vi "pll_proba_diag_realtime.vi"(0 "all rows":dbl[][](array[numeric])=array100002x3[300006 elements] format="%0.5f", 5 "Resolution":dbl, 7 "t_ref":dbl[](array[numeric]), 9 "dt":dbl, 11 "Error In":errorcluster, 12 "Second":bool) -> (3 "average":dbl=2.3596690204414683, 4 "XY Graph":cluster{"all rows":dbl[], "all rows":dbl[]}[](graph), 6 "Waveform Graph":cluster{"f0":dbl, "df":dbl, "magnitude":dbl[]}(graph), 8 "time":dbl[](array[numeric]), 10 "Waveform Graph 2":cluster{"f0":dbl, "df":dbl, "magnitude":dbl[]}(graph), 13 "PLL_sine":dbl[](array[numeric]), 14 "PLL_cosine":dbl[](array[numeric]), 15 "Error Out":errorcluster)   [LabVIEW 2013]
uses:
  <vilib>/express/express analysis/Spectral/Block/exnSpectralBlock spectral measurements RMS poly.vi
  <vilib>/express/express analysis/Spectral/Block/exnSpectralBlock spectral measurements RMS WFM.vi
  <vilib>/express/express analysis/Spectral/XNode/ExpressSpectralMeasurementsBlockNode.xnode
panel:
  out "XY Graph 2":cluster{"all rows":dbl[], "all rows":dbl[]}[](graph)
  out "t_i-1":dbl
  out "t_i":dbl
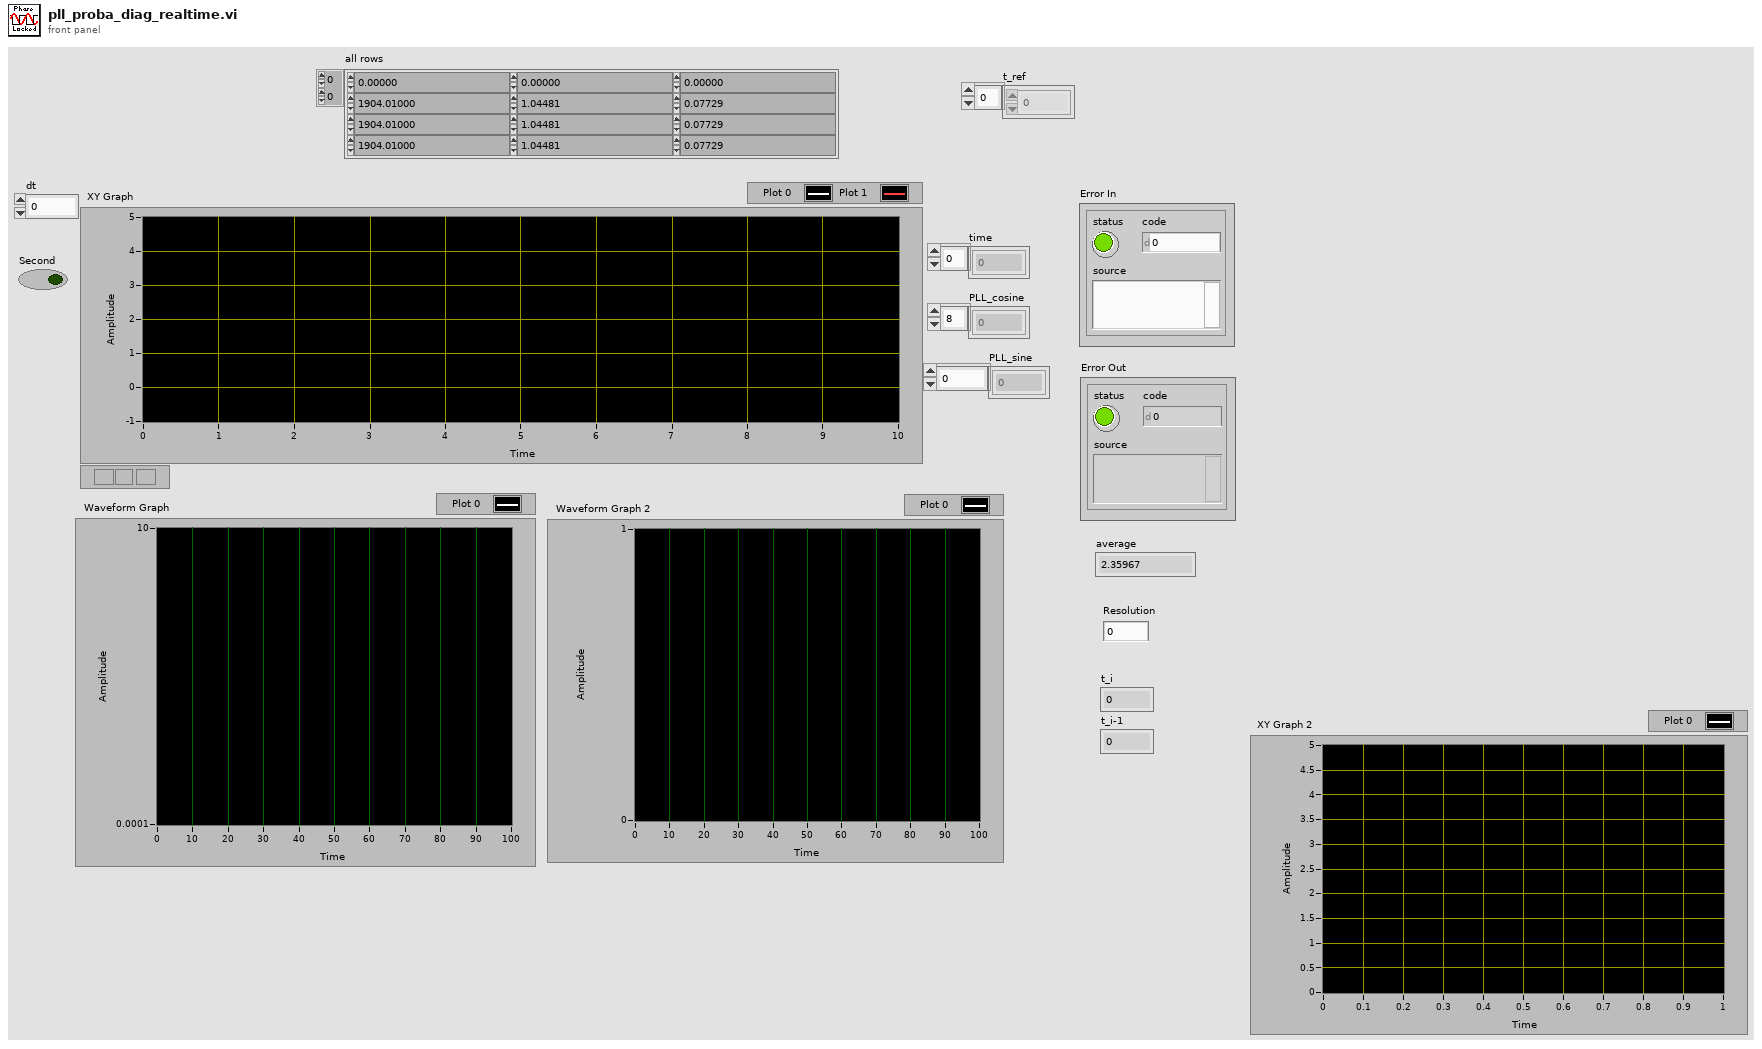
[diagram p1: front panel]
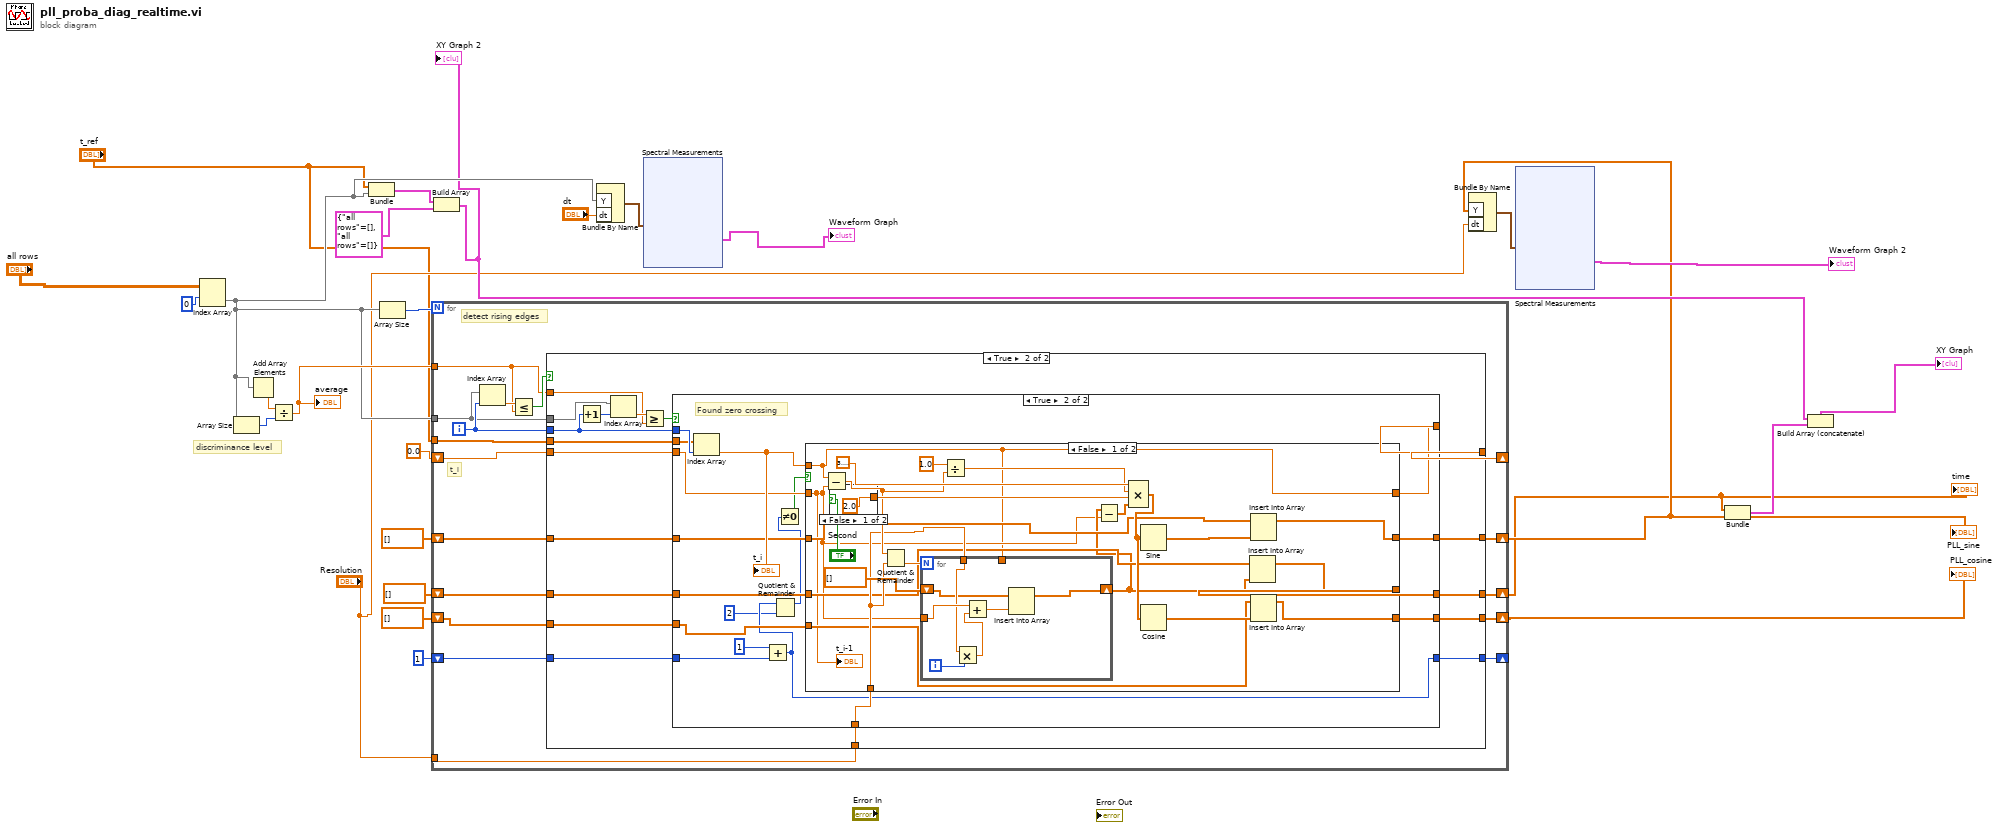
[diagram p0: block diagram]
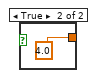
[diagram p4: hidden frame]
diagram:
  # "discriminance level"
  n1 = Index Array(array="all rows", index (row)=0 ("disabled index (col)")) -> (element=w19:dbl[])  [unwired: 1 in]
  n2 = Array Size(array=w19) -> (size(s)=w25:i32)
  n3 = Add Array Elements(numeric array=w19) -> (sum=w26:dbl)
  n4 = Divide(x=w26, y=w25) -> (x/y=w24:dbl)
  "average" <- w24
  n5 = Bundle("t_ref"="t_ref", "all rows"=w19) -> (w15:cluster{"t_ref":dbl[], "all rows":dbl[]})  [unwired: 1 in]
  n6 = Array Size(array=w19) -> (size(s)=w23:i32)
  n7 = for {
    N: w23 -> [_]
    tunnel: w19 -> [w42]
    tunnel: w24 -> [w40]
    tunnel: "t_ref" -> [w39]
    shift-right: [w38] -> _
    shift-left: 0.0 -> [w37]
    tunnel: "Resolution" -> [w36]
    shift-right: [w35] -> w5
    shift-left: dbl[] [] -> [w34]
    shift-right: [w33] -> w4
    shift-left: dbl[] [] -> [w32]
    shift-right: [w31] -> w3
    shift-left: dbl[] [] -> [w30]
    shift-right: [w29] -> _
    shift-left: 1 -> [w28]
    i -> [w43]
    # "t_i"
    # "detect rising edges"
    n8 = Index Array(array=w42, index=w43) -> (element=w41:dbl)
    n9 = Less Or Equal?(x=w41, y=w40) -> (x <= y?=w44:bool)
    n10 = case shown="True" w44 {
      tunnel: w43 -> [_ w61]
      tunnel: w42 -> [_ w67]
      tunnel: w40 -> [_ w63]
      tunnel: w39 -> [_ w62]
      tunnel: [w49 w60] -> w38
      tunnel: w37 -> [w49 w59]
      tunnel: w36 -> [_ w58]
      tunnel: [w48 w57] -> w35
      tunnel: w34 -> [w48 w56]
      tunnel: [w47 w55] -> w33
      tunnel: w32 -> [w47 w54]
      tunnel: [w46 w53] -> w31
      tunnel: w30 -> [w46 w52]
      tunnel: [w45 w51] -> w29
      tunnel: w28 -> [w45 w50]
      frame False {
      }
      frame True {
        n11 = Increment(x=w61) -> (x+1=w66:i32)
        n12 = Index Array(array=w67, index=w66) -> (element=w64:dbl)
        n13 = Greater Or Equal?(x=w64, y=w63) -> (x >= y?=w65:bool)
        n14 = case shown="True" w65 {
          tunnel: w62 -> [_ w89]
          tunnel: w61 -> [_ w90]
          tunnel: [w72 w73] -> w60
          tunnel: w59 -> [w72 w86]
          tunnel: w58 -> [_ w87]
          tunnel: [w71 w85] -> w57
          tunnel: w56 -> [w71 w82]
          tunnel: [w70 w84] -> w55
          tunnel: w54 -> [w70 w81]
          tunnel: [w69 w83] -> w53
          tunnel: w52 -> [w69 w80]
          tunnel: [w68 w77] -> w51
          tunnel: w50 -> [w68 w78]
          frame False {
          }
          frame True {
            # "Found zero crossing"
            n15 = Index Array(array=w89, index=w90) -> (element=w88:dbl)
            "t_i" <- w88
            n16 = Add(x=1, y=w78) -> (x+y=w77:i32)
            n17 = Quotient & Remainder(x=w77, y=2) -> (x-y*floor(x/y)=w74:i32)  [unwired: 1 out]
            n18 = Not Equal To 0?(x=w74) -> (x != 0?=w75:bool)
            n19 = case shown="False" w75 {
              tunnel: w86 -> [w92 w122]
              tunnel: w88 -> [w91 _]
              tunnel: w87 -> [w105 _]
              tunnel: [w97 w124] -> w84
              tunnel: [w100 w125] -> w85
              tunnel: [w94 w123] -> w83
              tunnel: w82 -> [w102 w125]
              tunnel: w81 -> [w99 w124]
              tunnel: w80 -> [w95 w123]
              tunnel: [w91 w122] -> w73
              frame False {
                n20 = Subtract(x=w91, y=w92) -> (x-y=w106:dbl)
                n21 = case shown="False" "Second" {
                  tunnel: [2.0 ("value") 4.0 ("value")] -> w111
                  frame False {
                  }
                  frame True {
                  }
                }
                n22 = Quotient & Remainder(x=w106, y=w105) -> (floor(x/y)=w104:dbl)  [unwired: 1 out]
                n23 = for {
                  N: w104 -> [_]
                  tunnel: w105 -> [w119]
                  tunnel: w92 -> [w120]
                  tunnel: w91 -> [_]
                  shift-right: [w121] -> w98
                  shift-left: dbl[] [] -> [w115]
                  i -> [w117]
                  n24 = Multiply(x=w119, y=w117) -> (x*y=w118:dbl)
                  n25 = Add(x=w120, y=w118) -> (x+y=w116:dbl)
                  n26 = Insert Into Array(array=w115, new element=w116) -> (w121:dbl[])  [unwired: 1 in]
                }
                n27 = Divide(x=1.0, y=w106) -> (x/y=w109:dbl)
                n28 = Subtract(x=w98, y=w92) -> (x-y=w107:dbl[])
                n29 = Compound Arithmetic op=MULTIPLY(3.141592653589793, w109, w111, w107) -> (w103:dbl[])
                n30 = Sine(x=w103) -> (sin(x)=w101:dbl[])
                n31 = Cosine(x=w103) -> (cos(x)=w96:dbl[])
                n32 = Insert Into Array(array=w99, new element=w98) -> (w97:dbl[])  [unwired: 1 in]
                n33 = Insert Into Array(array=w102, new element=w101) -> (w100:dbl[])  [unwired: 1 in]
                n34 = Insert Into Array(array=w95, new element=w96) -> (w94:dbl[])  [unwired: 1 in]
                "t_i-1" <- w92
              }
              frame True {
              }
            }
          }
        }
      }
    }
  }
  "PLL_sine" <- w5
  "PLL_cosine" <- w3
  "time" <- w4
  n35 = Build Array(w15, cluster{"all rows":dbl[], "all rows":dbl[]} {"all rows"=[], "all rows"=[]} ("element")) -> (w13:cluster{"all rows":dbl[], "all rows":dbl[]}[])
  "XY Graph 2" <- w13
  n36 = Bundle By Name("Y"=w19, "dt"="dt") -> (w20:waveform(dbl))  [unwired: 1 in]
  n37 = xnode "Spectral Measurements"("Signals"=w20) -> ("FFT - (RMS)"=→"Waveform Graph":cluster{"f0":dbl, "df":dbl, "magnitude":dbl[]})  [unwired: 1 in, 2 out]
  n38 = Bundle By Name("Y"=w5, "dt"="Resolution") -> (w17:waveform(dbl))  [unwired: 1 in]
  n39 = xnode "Spectral Measurements"("Signals"=w17) -> ("FFT - (RMS)"=→"Waveform Graph 2":cluster{"f0":dbl, "df":dbl, "magnitude":dbl[]})  [unwired: 1 in, 2 out]
  n40 = Bundle(w4, w5) -> (w21:cluster{dbl[], dbl[]})  [unwired: 1 in]
  n41 = Build Array (concatenate)(w13, w21) -> (→"XY Graph":cluster{"all rows":dbl[], "all rows":dbl[]}[])
